vi "Write States.vi"(8 "error in (no error)":errorcluster, 10 "States":enum16{"ZigZag", "Exit"}(ring), 11 "ZigZagTactic in":refnum<class "ZigZagTactic.lvclass">) -> (0 "error out":errorcluster, 3 "ZigZagTactic out":refnum<class "ZigZagTactic.lvclass">)   [LabVIEW 2023, in "ZigZagTactic.lvclass"]
uses:
  ZigZagTactic.lvclass
  ZigZagTactic.lvclass/ZigZagTactic.ctl
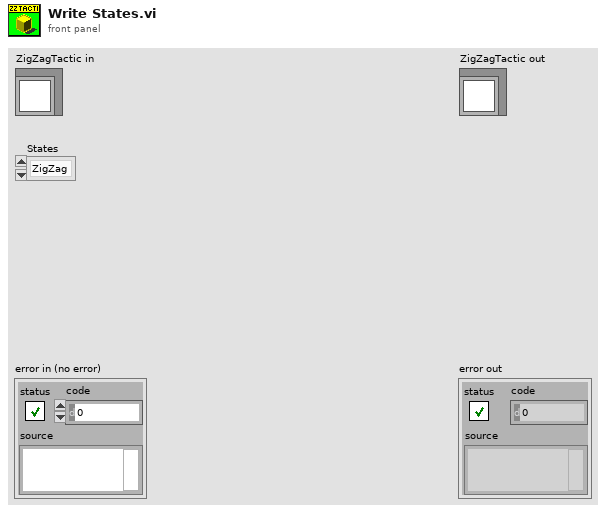
[diagram p1: front panel]
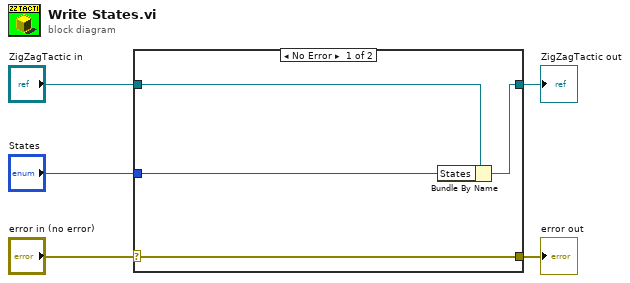
[diagram p0: block diagram]
diagram:
  n1 = case shown="No Error" "error in (no error)" {
    selector: "error in (no error)" -> [w9 w10]
    tunnel: [w9 w10] -> w4
    tunnel: [w7 w11] -> w2
    tunnel: "ZigZagTactic in" -> [w8 w11]
    tunnel: "States" -> [w6 _]
    frame No Error {
      n2 = Bundle By Name(cluster=w8, "States"=w6) -> (w7:refnum<class "ZigZagTactic.lvclass">)
    }
    frame Error {
    }
  }
  "error out" <- w4
  "ZigZagTactic out" <- w2
